vi "GetDataOneMeasurement.vi"   [LabVIEW 2013]
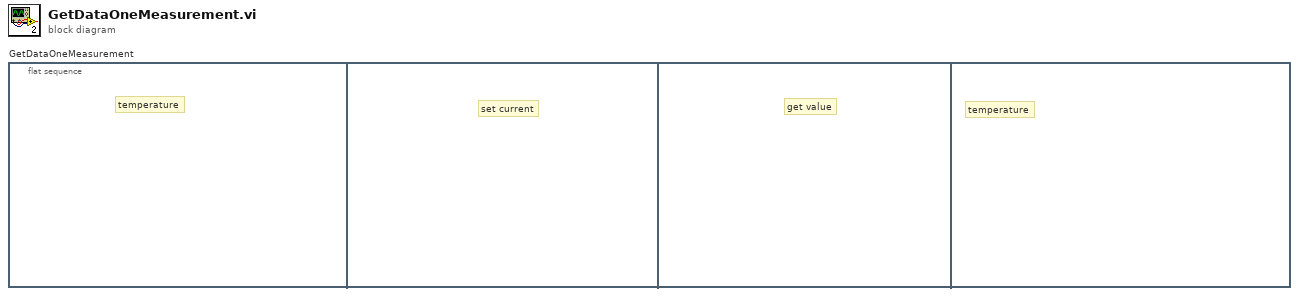
[diagram p0: block diagram]
diagram:
  n1 = flat-sequence "GetDataOneMeasurement" {
    frame #0 {
      # "temperature"
    }
    frame #1 {
      # "set current"
    }
    frame #2 {
      # "get value"
    }
    frame #3 {
      # "temperature"
    }
  }
